vi "getFrontPanelRef.vi"(8 "error in (no error)":errorcluster, 11 "ActionPanel in":refnum<class "playFileAction.lvclass">) -> (0 "error out":errorcluster, 2 "vi reference":refnum<vi>, 3 "ActionPanel out":refnum<class "playFileAction.lvclass">)   [LabVIEW 2011, in "Views.lvlib" / "ScriptEditor.lvlib" / "playFileAction.lvclass"]
uses:
  playFileAction.lvclass
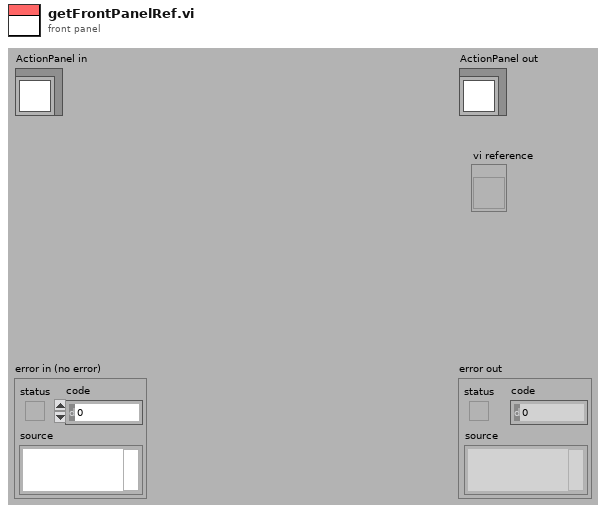
[diagram p1: front panel]
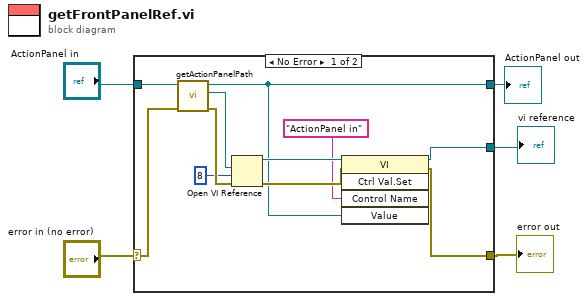
[diagram p0: block diagram]
diagram:
  n1 = case shown="No Error" "error in (no error)" {
    selector: "error in (no error)" -> [w15 w17]
    tunnel: "ActionPanel in" -> [w16 w18]
    tunnel: [w6 w17] -> w1
    tunnel: [w9 w18] -> w2
    tunnel: [w7 _] -> w3
    frame No Error {
      n2 = call-dynamic "getActionPanelPath.vi"("error in (no error)"=w15, "playFileAction in"=w16) -> ("error out"=w13:errorcluster, "frontPanelPath"=w14:path, "playFileAction out"=w9:refnum<class "playFileAction.lvclass">)  [unwired: 7 in]
      n3 = Open VI Reference(vi path=w14, options=8, error in (no error)=w13) -> (vi reference=w11:refnum<vi>, error out=w10:errorcluster)  [unwired: 3 in]
      n4 = invoke class="VI" method="Ctrl Val.Set"(reference=w11, error in=w10, "Control Name"="ActionPanel in", "Value"=w9) -> (reference out=w7:refnum<vi>, error out=w6:errorcluster)  [unwired: 1 in, 3 out]
    }
    frame Error {
    }
  }
  "error out" <- w1
  "ActionPanel out" <- w2
  "vi reference" <- w3
